vi "sub_main_ycar.vi"(8 "error in":errorcluster) -> (0 "error out":errorcluster)   [LabVIEW 2019]
uses:
  Ctrl/cmd_common.ctl
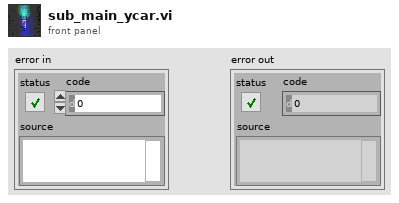
[diagram p1: front panel]
types:
  T1 = typedef "cmd_common.ctl" = enum16{"read", "write"}
  T2 = typedef "status.ctl" = u16
  T3 = cluster{"AGV":T2, "AGV Estop":T2, "Obstacle":T2, "Heading":T2, "Waypt":T2, "GNSS":T2, "VLP16":T2, "Cam":T2, "RPLidar":T2, "Joystick":T2}
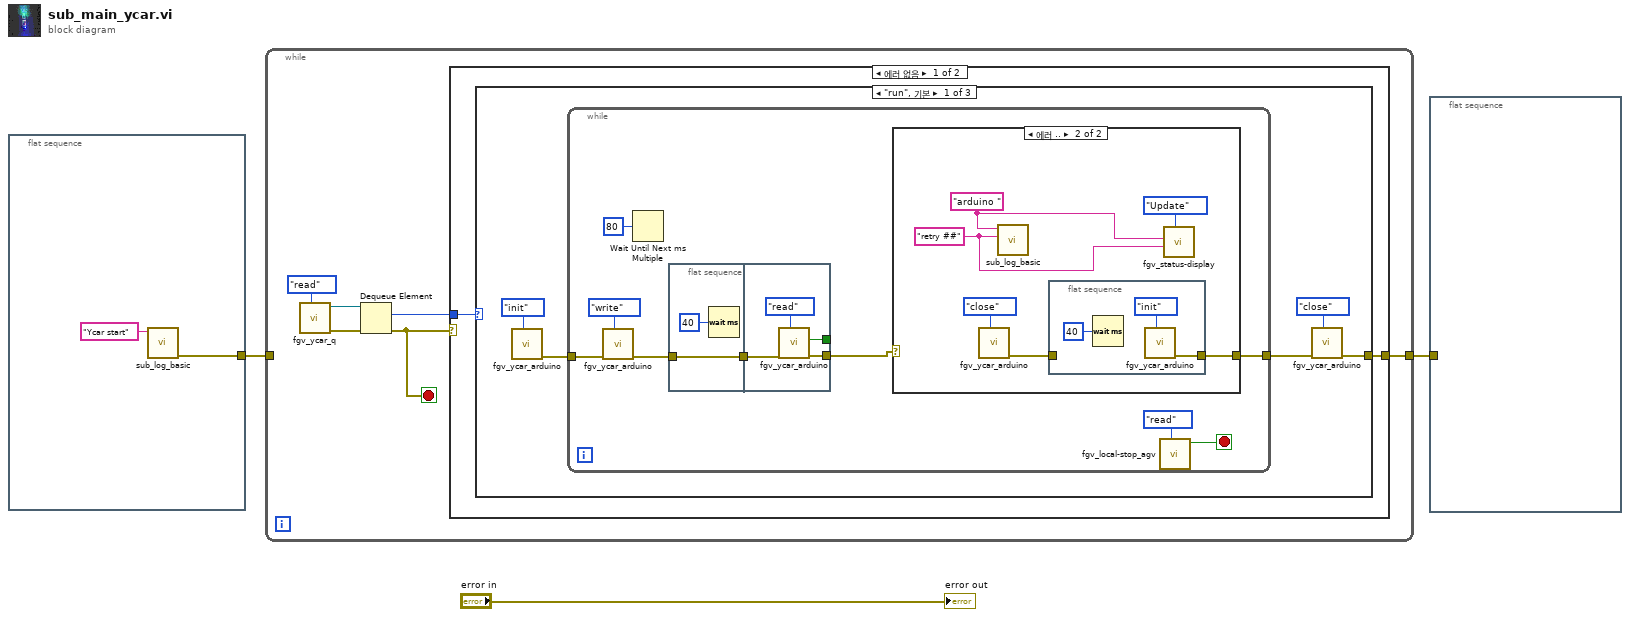
[diagram p0: block diagram]
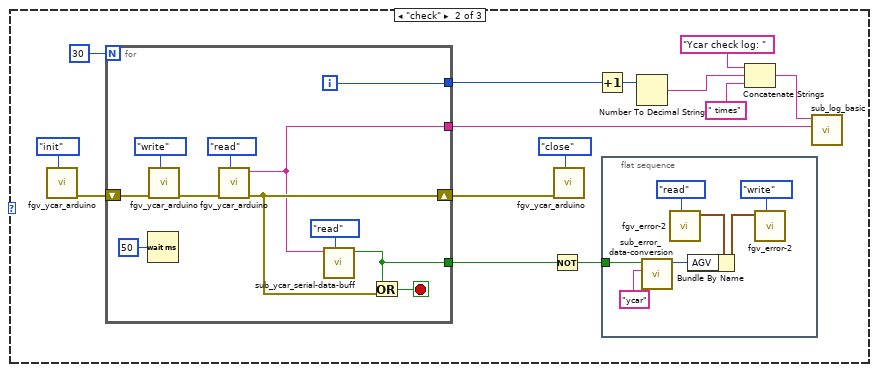
[diagram p3: hidden frame]
diagram:
  n1 = flat-sequence {
    tunnel: [w4] -> w1
    frame #0 {
      n2 = call "sub_log_basic.vi"("Title"="Ycar start") -> ("error out"=w4:errorcluster)  [unwired: 10 in]
    }
  }
  n3 = while {
    tunnel: [w7] -> w3
    tunnel: w1 -> [_]
    stop <- w6 stop-if-true
    n4 = call "fgv_ycar_q.vi"("cmd"=enum16{"create", "write", "read", "close"}."read") -> ("error out"=w10:errorcluster, "queue out"=w9:refnum<queue>)  [unwired: 9 in]
    n5 = Dequeue Element(queue=w9, error in (no error)=w10) -> (element=w8:enum16{"run", "check", "stop"}, error out=w6:errorcluster)  [unwired: 1 in, 2 out]
    n6 = case shown="에러 없음" w6 {
      tunnel: w8 -> [w13 _]
      tunnel: [w12 _] -> w7
      frame No Error {
        n7 = case shown="\"run\", 기본" w13 {
          tunnel: [w14 _ _] -> w12
          frame "run", Default {
            n8 = call "fgv_ycar_arduino.vi"("cmd"=enum16{"init", "read", "write", "close"}."init") -> ("error out"=w16:errorcluster)  [unwired: 8 in, 2 out]
            n9 = while {
              tunnel: w16 -> [w23]
              tunnel: [w20] -> w15
              stop <- w26 stop-if-true
              n10 = call "fgv_ycar_arduino.vi"("cmd"=enum16{"init", "read", "write", "close"}."write", "error in"=w23) -> ("error out"=w24:errorcluster)  [unwired: 7 in, 2 out]
              n11 = Wait Until Next ms Multiple(millisecond multiple=u32 80 ("milliseconds to wait")) -> ()  [unwired: 1 out]
              n12 = flat-sequence {
                tunnel: w24 -> [w38]
                tunnel: [w38] -> w21
                tunnel: [w40] -> w19
                tunnel: w21 -> [w41]
                tunnel: [w39] -> _
                frame #0 {
                  n13 = Wait (ms)(milliseconds to wait=u32 40) -> ()  [unwired: 1 out]
                }
                frame #1 {
                  n14 = call "fgv_ycar_arduino.vi"("cmd"=enum16{"init", "read", "write", "close"}."read", "error in"=w41) -> ("error out"=w40:errorcluster, "val"=w39:bool)  [unwired: 7 in, 1 out]
                }
              }
              n15 = case shown="에러 .." w19 {
                tunnel: [_ w31] -> w20
                frame No Error {
                }
                frame Error {
                  w28 = "retry ##" ("desc")
                  w29 = "arduino " ("Title")
                  n16 = call "fgv_ycar_arduino.vi"("cmd"=enum16{"init", "read", "write", "close"}."close") -> ("error out"=w32:errorcluster)  [unwired: 8 in, 2 out]
                  n17 = call "sub_log_basic.vi"("desc"=w28, "Title"=w29) -> ()  [unwired: 9 in, 1 out]
                  n18 = flat-sequence {
                    tunnel: w32 -> [_]
                    tunnel: [w35] -> w31
                    frame #0 {
                      n19 = Wait (ms)(milliseconds to wait=u32 40) -> ()  [unwired: 1 out]
                      n20 = call "fgv_ycar_arduino.vi"("cmd"=enum16{"init", "read", "write", "close"}."init") -> ("error out"=w35:errorcluster)  [unwired: 8 in, 2 out]
                    }
                  }
                  n21 = call "fgv_status-display.vi"("Mode"=enum16{"Initial", "Update", "Clear"}."Update", "detail"=w28, "title"=w29) -> ()  [unwired: 8 in, 1 out]
                }
              }
              n22 = call "fgv_local-stop_agv.vi"("cmd"=enum16{"ini", "read", "stop"}."read") -> ("stop status"=w26:bool)  [unwired: 10 in]
            }
            n23 = call "fgv_ycar_arduino.vi"("cmd"=enum16{"init", "read", "write", "close"}."close", "error in"=w15) -> ("error out"=w14:errorcluster)  [unwired: 7 in, 2 out]
          }
          frame "check" {
            n24 = call "fgv_ycar_arduino.vi"("cmd"=enum16{"init", "read", "write", "close"}."init") -> ("error out"=w54:errorcluster)  [unwired: 8 in, 2 out]
            n25 = for {
              N: 30 -> [_]
              shift-right: [w68] -> w53
              shift-left: w54 -> [w71]
              tunnel: [w69] -> w45
              tunnel: [w65] -> w44
              tunnel: [w64] -> w43
              i -> [w69]
              stop <- w67 stop-if-true
              n26 = Wait (ms)(milliseconds to wait=u32 50) -> ()  [unwired: 1 out]
              n27 = call "fgv_ycar_arduino.vi"("cmd"=enum16{"init", "read", "write", "close"}."write", "error in"=w71) -> ("error out"=w70:errorcluster)  [unwired: 7 in, 2 out]
              n28 = call "fgv_ycar_arduino.vi"("cmd"=enum16{"init", "read", "write", "close"}."read", "error in"=w70) -> ("error out"=w68:errorcluster, "read_buffer"=w65:string)  [unwired: 7 in, 1 out]
              n29 = call "sub_ycar_serial-data-buff.vi"("cmd"=cmd_common."read", "data"=w65) -> ("val"=w64:bool)  [unwired: 8 in, 1 out]
              n30 = Or(x=w64, y=w68) -> (x .or. y?=w67:bool)
            }
            n31 = Not(x=w43) -> (.not. x?=w51:bool)
            n32 = call "fgv_ycar_arduino.vi"("cmd"=enum16{"init", "read", "write", "close"}."close", "error in"=w53) -> ()  [unwired: 7 in, 3 out]
            n33 = Increment(x=w45) -> (x+1=w48:i32)
            n34 = flat-sequence {
              tunnel: w51 -> [w58]
              frame #0 {
                n35 = call "sub_error_data-conversion.vi"("name"="ycar", "error status"=w58) -> ("error conversion out"=w63:T2)  [unwired: 8 in, 1 out]
                n36 = call "fgv_error-2.vi"("cmd"=enum16{"init", "read", "write"}."read") -> ("Error cluster out"=w62:T3)  [unwired: 9 in, 1 out]
                n37 = Bundle By Name(cluster=w62, "AGV"=w63) -> (w61:T3)
                n38 = call "fgv_error-2.vi"("cmd"=enum16{"init", "read", "write"}."write", "Error cluster"=w61) -> ()  [unwired: 8 in, 2 out]
              }
            }
            n39 = Number To Decimal String(number=w48) -> (decimal integer string=w49:string)  [unwired: 1 in]
            n40 = Concatenate Strings("Ycar check log: " ("Title"), w49, " times" ("문자열")) -> (w50:string)
            n41 = call "sub_log_basic.vi"("desc"=w44, "Title"=w50) -> ()  [unwired: 9 in, 1 out]
          }
          frame "stop" {
          }
        }
      }
      frame Error {
      }
    }
  }
  n42 = flat-sequence {
    tunnel: w3 -> [_]
    frame #0 {
    }
  }
  "error out" <- "error in"
